vi "Process and Save Data.vi"(7 "step#":u32, 8 "error in":errorcluster, 9 "New Data Channels":T2, 10 "X-Vars":T1[](array[typedef]), 11 "Scan Driver.lvclass in":refnum<class "Scan Driver.lvclass">) -> (0 "error out":errorcluster, 3 "Scan Driver.lvclass out":refnum<class "Scan Driver.lvclass">)   [LabVIEW 2017, in "Scan Driver.lvclass"]
doc: "(Deprecated) Given a new data point, generate one or more auxilliary data points from a secondary source, e.g. a modulator Instrument or an internal computation algorithm. Immediately write all data points to a temporay backup file."
uses:
  Scan Driver.lvclass
  Instruments/Utility Classes/Readable/Data Channels.ctl
  Instruments/Utility Classes/Readable/Data Channel.ctl
  Instruments/Utility Classes/Readable/Data Point.ctl
  Instruments/Utility Classes/Readable/Time.ctl
  Instruments/Utility Classes/Readable/X.ctl
  Scan Driver.lvclass/Scan Driver.ctl
  <vilib>/Utility/file.llb/Write To Spreadsheet File (DBL).vi
  Data Processing/Aux Data Source/Aux Data Source.lvclass
  File IO/File IO.lvclass
  Instruments/Utility Classes/Readable/Readable.lvclass
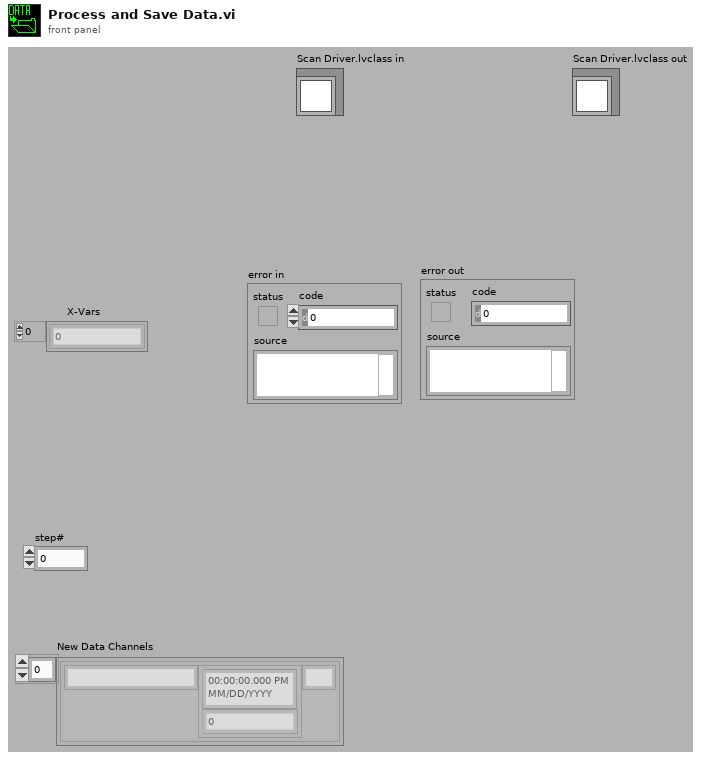
[diagram p1: front panel]
types:
  T1 = typedef "Readable.lvclass/X.ctl" = dbl
  T2 = typedef "Readable.lvclass/Data Channels.ctl" = T3[]
  T3 = typedef "Readable.lvclass/Data Channel.ctl" = cluster{"Name":string, "Data Point":T4, "Unit":string}
  T4 = typedef "Readable.lvclass/Data Point.ctl" = cluster{"t":T5, "x":T1}
  T5 = typedef "Readable.lvclass/Time.ctl" = timestamp
  T6 = typedef "Readable.lvclass/Data Store.ctl" = T4[][]
  T7 = cluster{"seconds since 1Jan1904":timestamp, "X-Var":T1}
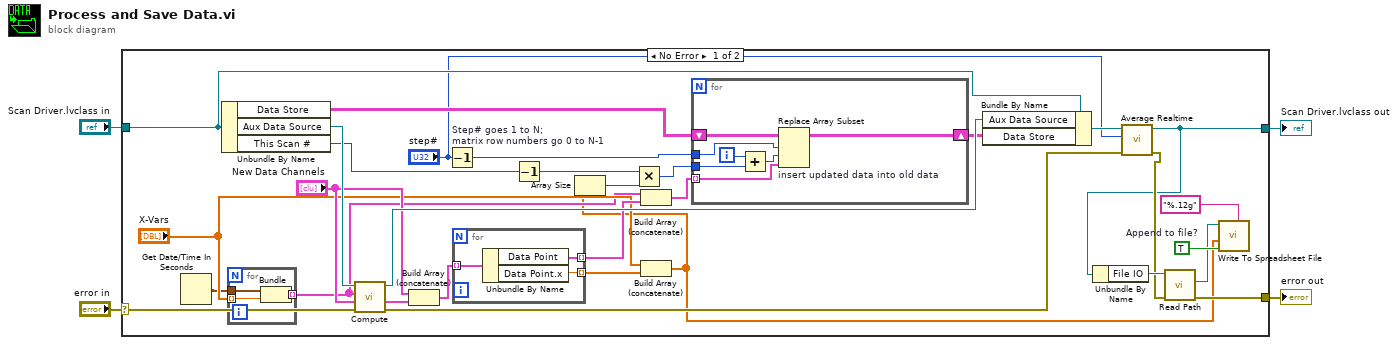
[diagram p0: block diagram]
diagram:
  n1 = case shown="No Error" "error in" {
    selector: "error in" -> [w24 w49]
    tunnel: [w23 w49] -> w3
    tunnel: "Scan Driver.lvclass in" -> [w33 w50]
    tunnel: [w11 w50] -> w1
    frame No Error {
      w34 = TRUE  # Append to file?
      n2 = Get Date/Time In Seconds() -> (seconds since 1Jan1904=w7:timestamp)
      n3 = Unbundle By Name(w33) -> ("Data Store"=w32:T6, "Aux Data Source"=w31:refnum<class "Aux Data Source.lvclass">, "This Scan #"=w17:u32)
      n4 = for {
        tunnel: "X-Vars" -> [w38] mode=indexing
        tunnel: w7 -> [w37]
        tunnel: [w36] -> w6 mode=indexing
        n5 = Bundle("seconds since 1Jan1904"=w37, "X-Var"=w38) -> (w36:T7)  [unwired: 1 in]
      }
      n6 = call-dynamic "Compute.vi"("error in (no error)"=w24, "Data Channels"="New Data Channels", "x-var"=w6, "Aux Data Source in"=w31) -> ("error out"=w13:errorcluster, "Add'l Data Channels"=w26:T2, "Aux Data Source out"=w27:refnum<class "Aux Data Source.lvclass">)  [unwired: 5 in]
      n7 = Build Array (concatenate)("New Data Channels", w26) -> (w25:T2)
      n8 = Decrement "Step# goes 1 to N;\nmatrix row numbers go 0 to N-1"(x="step#") -> (x-1=w10:u32)
      n9 = for {
        tunnel: w25 -> [w47] mode=indexing
        tunnel: [w48] -> w21 mode=indexing
        tunnel: [w46] -> w20 mode=indexing
        n10 = Unbundle By Name(w47) -> ("Data Point"=w46:T4, "Data Point.x"=w48:T1)
      }
      n11 = Decrement(x=w17) -> (x-1=w14:u32)
      n12 = Build Array (concatenate)(w6, w20) -> (w19:T4[])
      n13 = Build Array (concatenate)("X-Vars", w21) -> (w5:T1[])
      n14 = Array Size(array=w5) -> (size(s)=w15:i32)
      n15 = Multiply(x=w14, y=w15) -> (x*y=w16:u32)
      n16 = for {
        tunnel: w10 -> [w44]
        tunnel: w19 -> [w39] mode=indexing
        shift-right: [w43] -> w18
        shift-left: w32 -> [w45]
        tunnel: w16 -> [w40]
        i -> [w42]
        n17 = Add(x=w42, y=w40) -> (x+y=w41:u32)
        n18 = Replace Array Subset "insert updated data into old data"(array=w45, new element=w39, index (row)=w44, index (col)=w41) -> (w43:T6)
      }
      n19 = Bundle By Name(cluster=w33, "Aux Data Source"=w27, "Data Store"=w18) -> (w30:refnum<class "Scan Driver.lvclass">)
      n20 = call-dynamic "Average Realtime.vi"("error in"=w13, "Current Step"="step#", "Scan Driver.lvclass"=w30) -> ("error out"=w12:errorcluster, "Scan Driver.lvclass out"=w11:refnum<class "Scan Driver.lvclass">)  [unwired: 7 in]
      n21 = Unbundle By Name(w11) -> ("File IO"=w29:refnum<class "File IO.lvclass">)
      n22 = call-dynamic "Read Path.vi"("error in (no error)"=w12, "File IO.lvclass in"=w29) -> ("error out"=w23:errorcluster, "Temporary Path"=w28:path)  [unwired: 8 out]
      n23 = call-poly <vilib>:"Write To Spreadsheet File.vi"("format (%.3f)"="%.12g", "append to file? (new file:F)"=w34, "1D data"=w5, "file path (dialog if empty)"=w28) -> ()  [unwired: 2 in, 3 out]
    }
    frame Error {
    }
  }
  "Scan Driver.lvclass out" <- w1
  "error out" <- w3
